vi "Assert Log File Duration.vi"(8 "error in (no error)":errorcluster, 11 "Embedded Data Logger System Tests in":refnum<class "Embedded Data Logger System Tests.lvclass">) -> (0 "error out":errorcluster, 3 "Embedded Data Logger System Tests out":refnum<class "Embedded Data Logger System Tests.lvclass">)   [LabVIEW 2018, in "Embedded Data Logger System Tests.lvclass"]
uses:
  Embedded Data Logger System Tests.lvclass
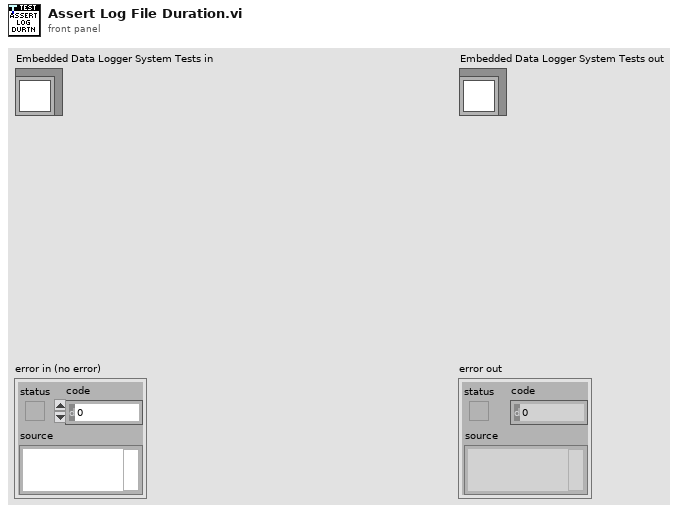
[diagram p1: front panel]
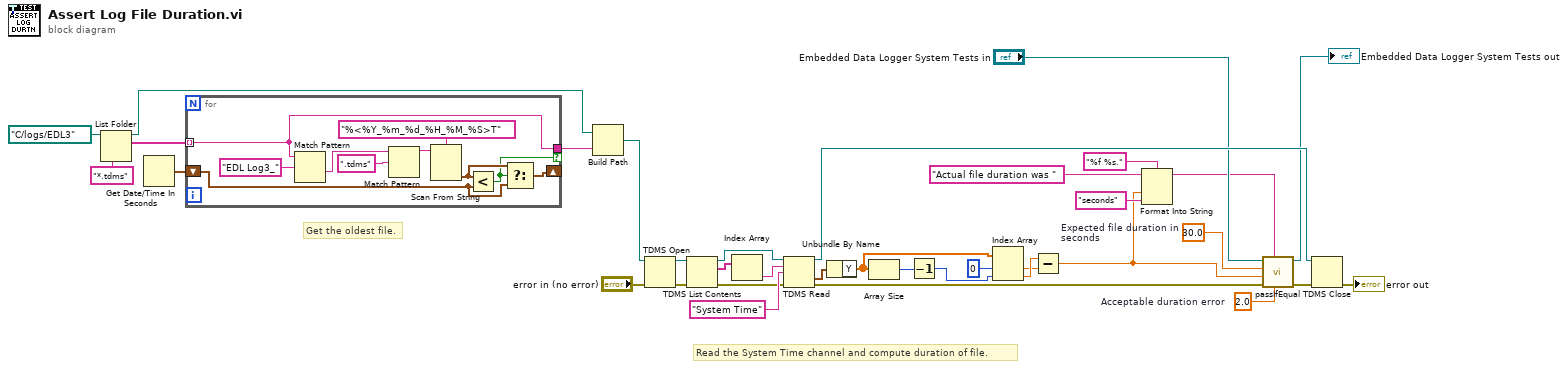
[diagram p0: block diagram]
diagram:
  w11 = 2.0  # Acceptable duration error
  w6 = 30.0  # Expected file duration in seconds
  # "Read the System Time channel and compute duration of file."
  # "Get the oldest file."
  n1 = List Folder(path=path "C:/logs/EDL3" ("file path"), pattern="*.tdms") -> (path out=w29:path, filenames=w32:string[])  [unwired: 2 in, 2 out]
  n2 = Get Date/Time In Seconds() -> (seconds since 1Jan1904=w31:timestamp)
  n3 = for {
    tunnel: w32 -> [w40] mode=indexing
    shift-right: [w41] -> _
    shift-left: w31 -> [w42]
    tunnel: [w40] -> w30 if=w39
    n4 = Match Pattern(string=w40, regular expression="EDL Log3_") -> (after substring=w38:string)  [unwired: 1 in, 3 out]
    n5 = Match Pattern(string=w38, regular expression=".tdms") -> (before substring=w36:string)  [unwired: 1 in, 3 out]
    n6 = Scan From String(format string="%<%Y_%m_%d_%H_%M_%S>T", input string=w36) -> (output 1=w43:timestamp)  [unwired: 3 in, 3 out]
    n7 = Less?(x=w43, y=w42) -> (x < y?=w39:bool)
    n8 = Select(t=w43, s=w39, f=w42) -> (s? t:f=w41:timestamp)
  }
  n9 = Build Path(base path=w29, name or relative path=w30) -> (appended path=w27:path)
  n10 = TDMS Open(8:"error in (no error)", 11:w27) -> (0:w34:errorcluster, 3:w35:refnum<k34>)  [unwired: 5 in]
  n11 = TDMS List Contents(4:w34, 7:w35) -> (0:w15:errorcluster, 2:w26:string[], 3:w25:refnum<k34>)  [unwired: 1 in, 1 out]
  n12 = Index Array(array=w26) -> (element=w24:string)  [unwired: 1 in]
  n13 = TDMS Read(0:w25, 5:w24, 7:"System Time", 11:w15) -> (4:w14:refnum<k34>, 10:w22:waveform(dbl), 15:w8:errorcluster)  [unwired: 4 in, 3 out]
  n14 = Unbundle By Name(w22) -> ("Y"=w21:dbl[])
  n15 = Array Size(array=w21) -> (size(s)=w20:i32)
  n16 = Decrement(x=w20) -> (x-1=w19:i32)
  n17 = Index Array(array=w21, index #1=0 ("index"), index #2=w19) -> (element #1=w16:dbl, element #2=w17:dbl)
  n18 = Subtract(x=w17, y=w16) -> (x-y=w2:dbl)
  n19 = Format Into String(format string="%f %s.", initial string="Actual file duration was ", w2, "seconds" ("input 2")) -> (resulting string=w1:string)  [unwired: 1 in, 1 out]
  n20 = call-dynamic "passIfEqual.vi"("delta (optional)"=w11, "custom report message (\"\")"=w1, "error in (no error)"=w8, "y"=w2, "x"=w6, "TestCase in"="Embedded Data Logger System Tests in") -> ("error out"=w7:errorcluster, "TestCase out"=→"Embedded Data Logger System Tests out":refnum<class "Embedded Data Logger System Tests.lvclass">)  [unwired: 4 in]
  n21 = TDMS Close(8:w7, 11:w14) -> (0:→"error out":errorcluster)  [unwired: 1 out]
